vi "Parse Dual Remote Terminal.vi"(8 "error in (no error)":errorcluster, 11 "Dual RT XML Node":refnum<k20>) -> (0 "error out":errorcluster, 3 "Dual RT":refnum<class "Remote Terminal.lvclass">[](array[class]))   [LabVIEW 2020]
uses:
  Remote Terminal/Remote Terminal.lvclass
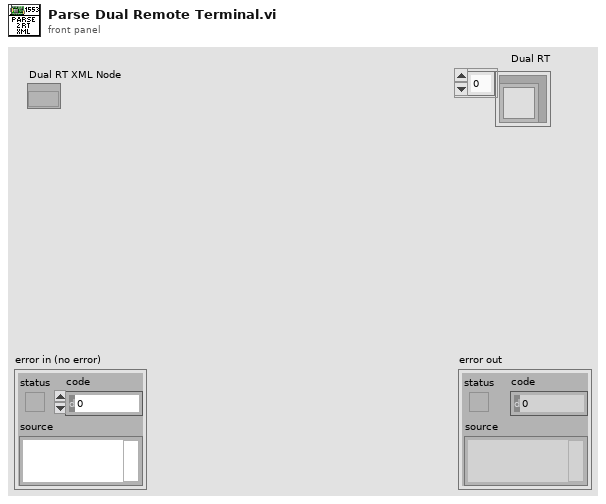
[diagram p1: front panel]
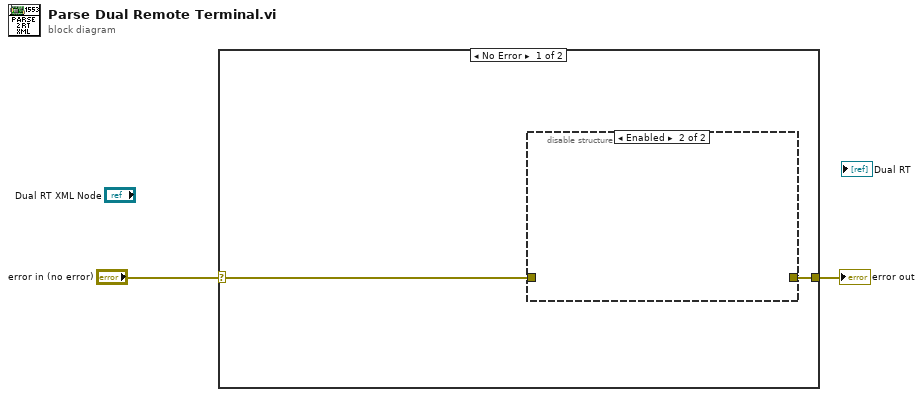
[diagram p0: block diagram]
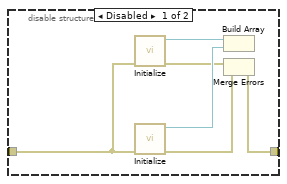
[diagram p2: hidden frame]
diagram:
  n1 = case shown="No Error" "error in (no error)" {
    selector: "error in (no error)" -> [w4 w11]
    tunnel: [w3 w11] -> w1
    frame No Error {
      n2 = disable-structure shown="Enabled" {
        disable-tunnel: w4 -> [w6 _]
        disable-tunnel: [w5 _] -> w3
        frame Disabled {
          n3 = call "Initialize.vi"("error in (no error)"=w6) -> ("error out"=w8:errorcluster, "Remote Terminal out"=w10:refnum<class "Remote Terminal.lvclass">)  [unwired: 9 in]
          n4 = call "Initialize.vi"("error in (no error)"=w6) -> ("error out"=w7:errorcluster, "Remote Terminal out"=w9:refnum<class "Remote Terminal.lvclass">)  [unwired: 9 in]
          n5 = Build Array(w10, w9) -> ()  [unwired: 1 out]
          n6 = Merge Errors(w8, w7) -> (w5:errorcluster)
        }
        frame Enabled {
        }
      }
    }
    frame Error {
    }
  }
  "error out" <- w1
